vi "ReadImageFileWithVisionInfo.vi"(6 "Use File Path Image Type":bool=TRUE, 7 "File Path":path, 8 "error in":errorcluster, 10 "Load Color Pallete":bool, 11 "Image Reference In":T2) -> (0 "error out":errorcluster, 3 "Image Reference Out":T2, 5 "Color Palette":T1[](array[typedef]))   [LabVIEW 2024, in "OpenLvVision_Image.lvlib" / "File.lvlib"]
doc: "Reads an image and the vision info saved allong ( Overlays, custom data)"
uses:
  File.lvlib
  Management/TypeDef/Image.ctl
  TypeDef/ColorPaletteValue.ctl
  Management/Management.lvlib
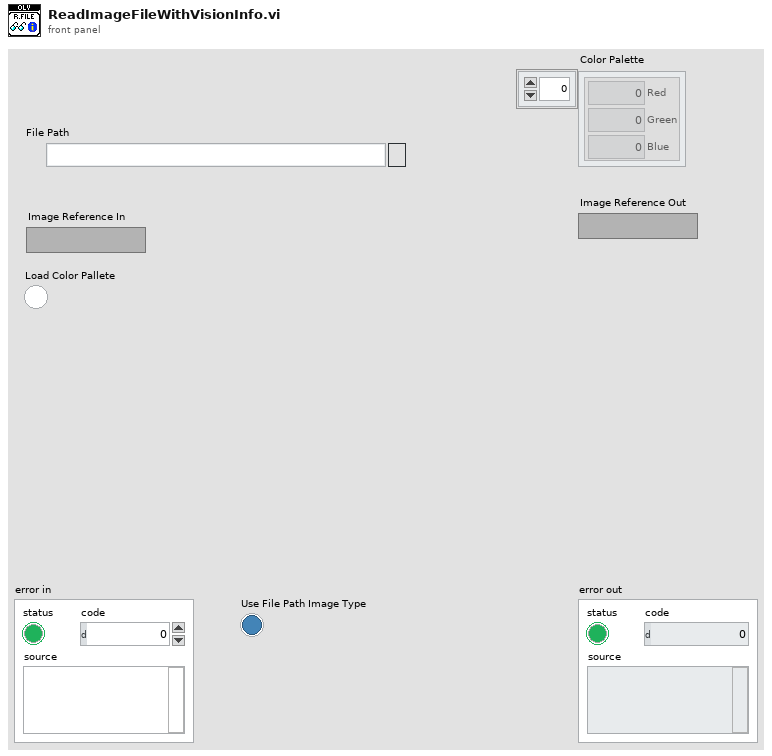
[diagram p1: front panel]
types:
  T1 = typedef "OpenLvVision_Image.lvlib/File.lvlib/ColorPaletteValue.ctl" = cluster{"Red":u8, "Green":u8, "Blue":u8}
  T2 = typedef "OpenLvVision_Image.lvlib/Management.lvlib/Image.ctl" = refnum<image>
  T3 = typedef "IMAQ Image.ctl" = refnum<image>
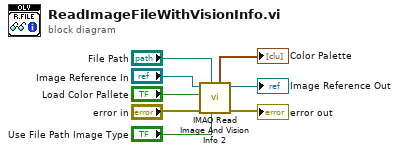
[diagram p0: block diagram]
diagram:
  n1 = call "IMAQ Read Image And Vision Info 2"("Use File Path Image Type"="Use File Path Image Type", "File Path"="File Path", "error in (no error)"="error in", "Load Color Palette? (No)"="Load Color Pallete", "Image"="Image Reference In") -> ("error out"=→"error out":errorcluster, "Image Out"=→"Image Reference Out":T3, "Color Palette out"=→"Color Palette":cluster{"Red":u8, "Green":u8, "Blue":u8}[])  [unwired: 4 in]
